vi "Call Dialog.vi"(8 "error in":errorcluster, 10 "Dialog":T1, 11 "Master Controller in":refnum<class "EMS User Interface.lvclass">) -> (0 "error out":errorcluster, 3 "Master Controller out":refnum<class "EMS User Interface.lvclass">)   [LabVIEW 2018, in "EMS User Interface Actor.lvlib" / "EMS User Interface.lvclass"]
uses:
  EMS User Interface.lvclass
  Controls/Dialog Message Selector.ctl
  Dialog VIs/Optimization Selection.vi
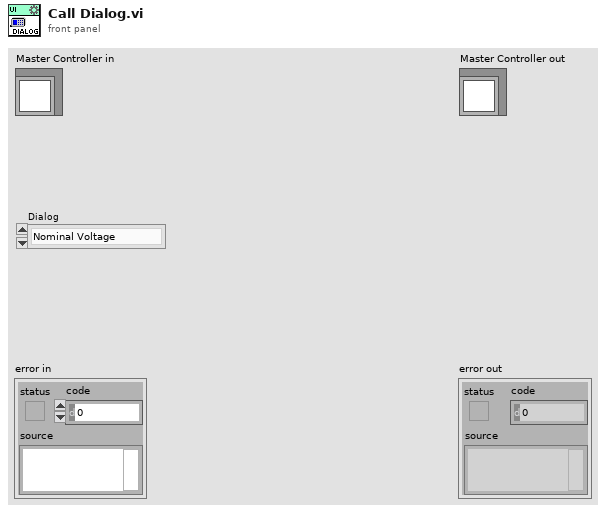
[diagram p1: front panel]
types:
  T1 = typedef "EMS User Interface Actor.lvlib/EMS User Interface.lvclass/Dialog Message Selector.ctl" = enum16{"Nominal Voltage", "Nominal Frequency", "Optimization Parameters"}
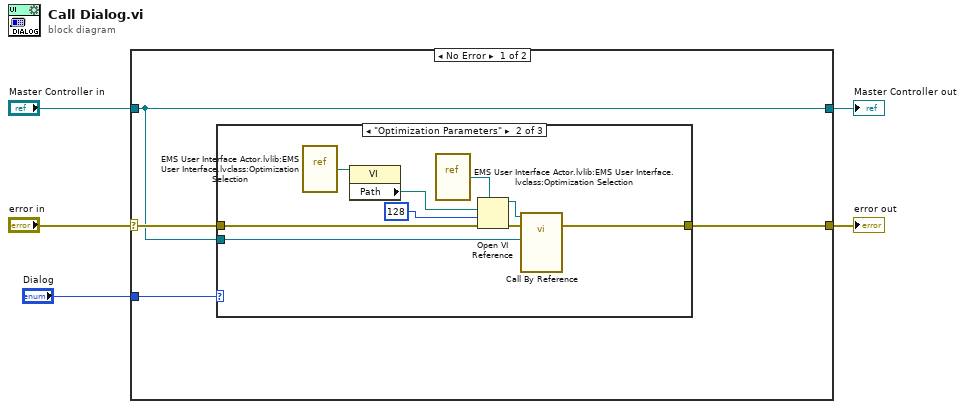
[diagram p0: block diagram]
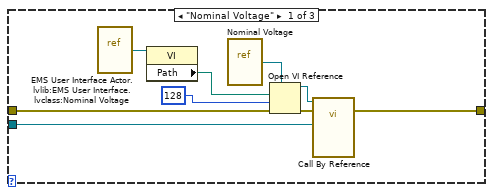
[diagram p2: hidden frame]
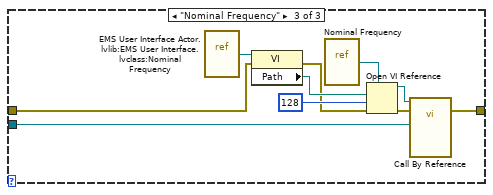
[diagram p3: hidden frame]
diagram:
  n1 = case shown="No Error" "error in" {
    selector: "error in" -> [w9 w39]
    tunnel: [w8 w39] -> w4
    tunnel: [w7 w38] -> w2
    tunnel: "Master Controller in" -> [w7 w38]
    tunnel: "Dialog" -> [w6 _]
    frame No Error {
      n2 = case shown="\"Optimization Parameters\"" w6 {
        tunnel: w9 -> [w13 w22 w28]
        tunnel: [w14 w23 w33] -> w8
        tunnel: w7 -> [w12 w21 w32]
        frame "Nominal Voltage" {
          n3 = vi-ref "EMS User Interface Actor.lvlib:EMS User Interface.lvclass:Nominal Voltage.vi"() -> (w11:refnum<vi>)
          n4 = property class="VI"(reference=w11) -> ("Path"=w10:path)  [unwired: 1 in, 2 out]
          n5 = vi-ref "Nominal Voltage.vi"() -> (w18:refnum<vi>)
          n6 = Open VI Reference(type specifier VI Refnum (for type only)=w18, vi path=w10, options=128, error in (no error)=w13) -> (vi reference=w17:refnum<vi>, error out=w16:errorcluster)  [unwired: 2 in]
          n7 = call-by-ref "?"(reference=w17, error in=w16, "Master Controller in"=w12) -> (error out=w14:errorcluster)  [unwired: 11 in, 1 out]
        }
        frame "Optimization Parameters" {
          n8 = vi-ref "EMS User Interface Actor.lvlib:EMS User Interface.lvclass:Optimization Selection.vi"() -> (w20:refnum<vi>)
          n9 = property class="VI"(reference=w20) -> ("Path"=w19:path)  [unwired: 1 in, 2 out]
          n10 = vi-ref "EMS User Interface Actor.lvlib:EMS User Interface.lvclass:Optimization Selection.vi"() -> (w27:refnum<vi>)
          n11 = Open VI Reference(type specifier VI Refnum (for type only)=w27, vi path=w19, options=128, error in (no error)=w22) -> (vi reference=w26:refnum<vi>, error out=w25:errorcluster)  [unwired: 2 in]
          n12 = call-by-ref "?"(reference=w26, error in=w25, "Master Controller in"=w21) -> (error out=w23:errorcluster)  [unwired: 11 in, 1 out]
        }
        frame "Nominal Frequency" {
          n13 = vi-ref "EMS User Interface Actor.lvlib:EMS User Interface.lvclass:Nominal Frequency.vi"() -> (w31:refnum<vi>)
          n14 = property class="VI"(reference=w31, error in=w28) -> (error out=w29:errorcluster, "Path"=w30:path)  [unwired: 1 out]
          n15 = vi-ref "Nominal Frequency.vi"() -> (w37:refnum<vi>)
          n16 = Open VI Reference(type specifier VI Refnum (for type only)=w37, vi path=w30, options=128, error in (no error)=w29) -> (vi reference=w36:refnum<vi>, error out=w35:errorcluster)  [unwired: 2 in]
          n17 = call-by-ref "?"(reference=w36, error in=w35, "Master Controller in"=w32) -> (error out=w33:errorcluster)  [unwired: 11 in, 1 out]
        }
      }
    }
    frame Error {
    }
  }
  "error out" <- w4
  "Master Controller out" <- w2
